vi "iRobot Open.vi"(8 "error in (no error)":errorcluster, 11 "UART port in":T1) -> (0 "error out":errorcluster, 3 "UART port out":T1)   [LabVIEW 2013]
doc: "Open UART serial port and initilize iRobot."
uses:
  Advanced/UART/iRobot UART Port Type.ctl
  Actuator/LED.ctl
  Advanced/Command/Baud.ctl
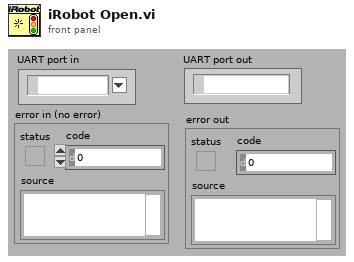
[diagram p1: front panel]
types:
  T1 = typedef "iRobot UART Port Type.ctl" = refnum<visa-resource-name>
  T2 = typedef "LED.ctl" = u8
  T3 = typedef "Baud.ctl" = enum8{"300", "600", "1200", "2400", "4800", "9600", "14400", "19200", "28800", "38400", "57600", "115200"}
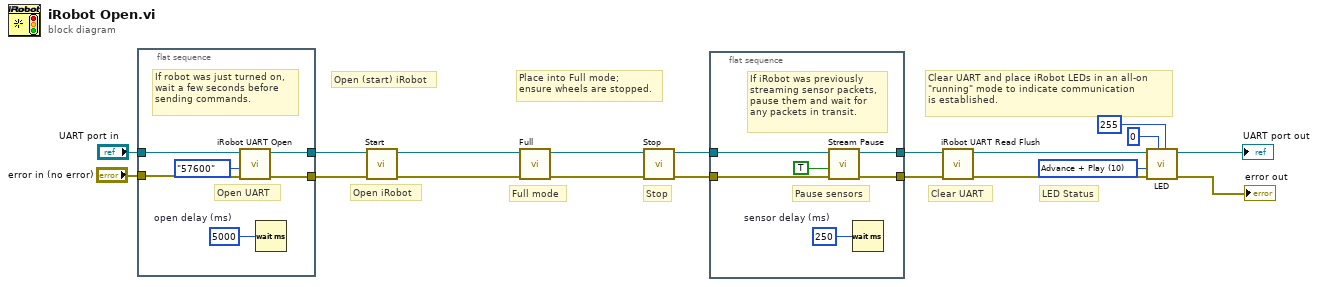
[diagram p0: block diagram]
diagram:
  w5 = T2 10 items=["None"=0, "Advance"=8, "Play"=2, "Advance + Play"=10] ("LEDs on")
  # "Clear UART and place iRobot LEDs in an all-on\n\"running\" mode to indicate communication\nis established."
  # "Clear UART"
  # "LED Status"
  # "Place into Full mode;\nensure wheels are stopped."
  # "Full mode"
  # "Stop"
  # "Open (start) iRobot"
  # "Open iRobot"
  n1 = flat-sequence {
    tunnel: "UART port in" -> [w25]
    tunnel: [w24] -> w12
    tunnel: [w23] -> w10
    tunnel: "error in (no error)" -> [w20]
    frame #0 {
      w22 = u32 5000  # open delay (ms)
      # "If robot was just turned on,\nwait a few seconds before\nsending commands."
      # "Open UART"
      n2 = call "iRobot UART Open.vi"("error in (no error)"=w20, "Baud Rate (BPS)"=Baud."57600", "UART port in"=w25) -> ("error out"=w23:errorcluster, "UART port out"=w24:T1)  [unwired: 7 out]
      n3 = Wait (ms)(milliseconds to wait=w22) -> ()  [unwired: 1 out]
    }
  }
  n4 = call "Start.vi"("error in"=w10, "UART port in"=w12) -> ("error out"=w9:errorcluster, "UART port out"=w11:T1)  [unwired: 8 out]
  n5 = call "Full.vi"("error in"=w9, "UART port in"=w11) -> ("error out"=w7:errorcluster, "UART port out"=w8:T1)  [unwired: 8 out]
  n6 = call "Stop.vi"("error in"=w7, "UART port in"=w8) -> ("error out"=w15:errorcluster, "UART port out"=w17:T1)  [unwired: 8 out]
  n7 = flat-sequence {
    tunnel: [w31] -> w19
    tunnel: w17 -> [w30]
    tunnel: w15 -> [w29]
    tunnel: [w28] -> w14
    frame #0 {
      w27 = u32 250  # sensor delay (ms)
      # "If iRobot was previously\nstreaming sensor packets,\npause them and wait for\nany packets in transit."
      # "Pause sensors"
      n8 = call "Stream Pause.vi"("error in"=w29, "Pause?"=TRUE ("Resume?"), "UART port in"=w30) -> ("error out"=w28:errorcluster, "UART port out"=w31:T1)  [unwired: 1 in, 6 out]
      n9 = Wait (ms)(milliseconds to wait=w27) -> ()  [unwired: 1 out]
    }
  }
  n10 = call "iRobot UART Read Flush.vi"("error in"=w14, "UART port in"=w19) -> ("error out"=w4:errorcluster, "UART port out"=w6:T1)  [unwired: 8 out]
  n11 = call "LED.vi"("Power LED Intensity (0-255)"=u8 255 ("Power LED Color (R-G)"), "Power LED Color (G[0]-R[255])"=u8 0, "error in"=w4, "LEDs on"=w5, "UART port in"=w6) -> ("error out"=→"error out":errorcluster, "UART port out"=→"UART port out":T1)  [unwired: 3 in, 2 out]
